vi "worksheet write url opt.vi"(4 "tooltip":string, 5 "string":string, 6 "format":u32, 7 "url":string, 8 "error in (no error)":errorcluster, 9 "col":u16, 10 "row":u32, 11 "worksheet":u32) -> (0 "error out":errorcluster, 3 "function return":u32(ring))   [LabVIEW 8.6]
doc: "lxw_error worksheet_write_url_opt(lxw_worksheet worksheet, lxw_row_t row, lxw_col_t col, const char *url, lxw_format format, const char *string, const char *tooltip);"
uses:
  pending_lvxlsxwriter/xlsxwriter.dll
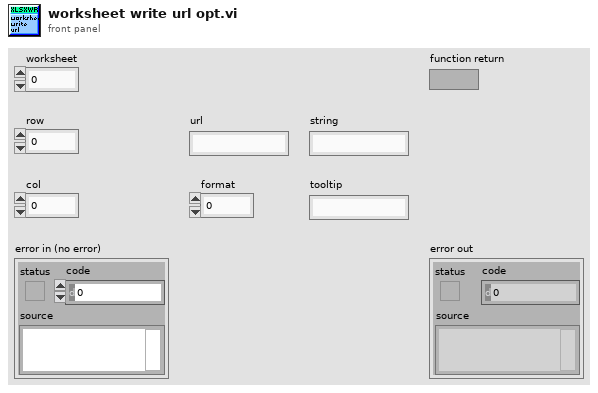
[diagram p1: front panel]
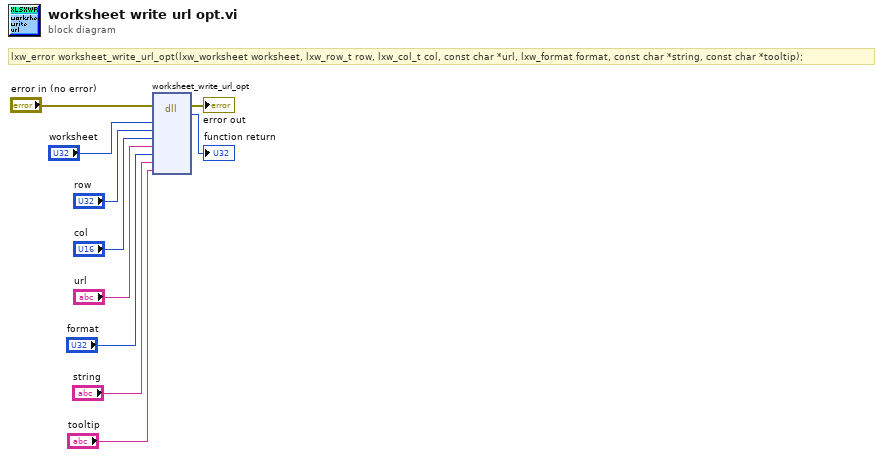
[diagram p0: block diagram]
diagram:
  # "lxw_error worksheet_write_url_opt(lxw_worksheet worksheet, lxw_row_t row, lxw_col_t col, const char *url, lxw_format format, const char *string, const char *tooltip);"
  n1 = dll-call lib="C:/Users/WDAGUtilityAccount/Desktop/pending_lvxlsxwriter/xlsxwriter.*" fn="worksheet_write_url_opt"(error in="error in (no error)", "worksheet"="worksheet", "row"="row", "col"="col", "url"="url", "format"="format", "string"="string", "tooltip"="tooltip") -> (error out=→"error out":errorcluster, →"function return":u32)  [unwired: 9 in, 1 out]
